vi "Send Request.vi"(8 "error in (no error)":errorcluster, 10 "ServerRequest":refnum<class "ControlPacket.lvclass">, 11 "Session in":refnum<class "Session.lvclass">) -> (0 "error out":errorcluster, 3 "Session out":refnum<class "Session.lvclass">)   [LabVIEW 2013, in "MQTT Server.lvlib" / "Session.lvclass"]
uses:
  Session.lvclass
  Control Packets/ControlPacket/ControlPacket.lvclass
  Server class/Request -- cluster.ctl
  Server class/Response -- cluster.ctl
  Session.lvclass/Session.ctl
  Server class/Server.lvclass
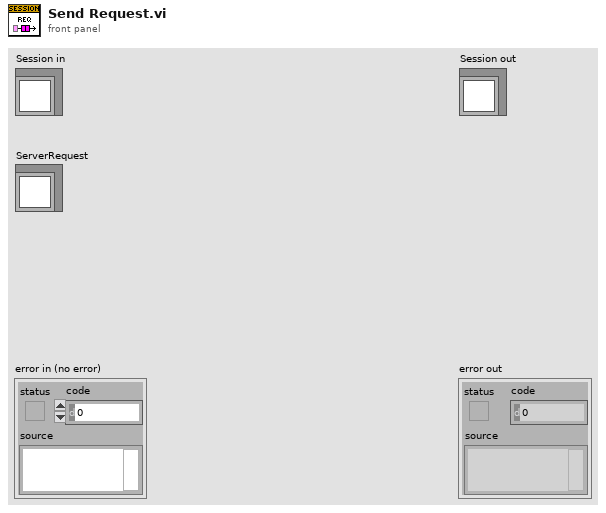
[diagram p1: front panel]
types:
  T1 = typedef "MQTT Server.lvlib/Server.lvclass/Request -- cluster.ctl" = cluster{"ServerRequest":refnum<class "ControlPacket.lvclass">, "SessionMailbox":refnum<queue>}
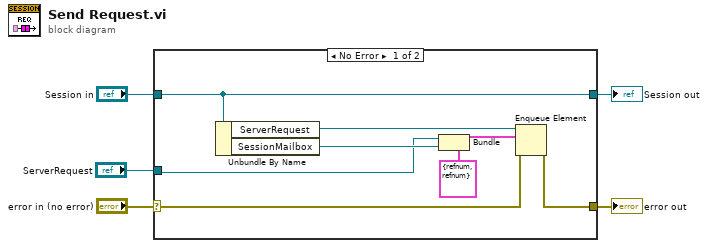
[diagram p0: block diagram]
diagram:
  n1 = case shown="No Error" "error in (no error)" {
    selector: "error in (no error)" -> [w11 w15]
    tunnel: [w10 w15] -> w4
    tunnel: [w13 w14] -> w2
    tunnel: "Session in" -> [w13 w14]
    tunnel: "ServerRequest" -> [w8 _]
    frame No Error {
      n2 = Unbundle By Name(w13) -> ("ServerRequest"=w12:refnum<queue>, "SessionMailbox"=w9:refnum<queue>)
      n3 = Bundle(cluster=T1 {"ServerRequest"=refnum, "SessionMailbox"=refnum} ("Request"), "ServerRequest"=w8, "SessionMailbox"=w9) -> (w7:T1)
      n4 = Enqueue Element(queue=w12, element=w7, error in (no error)=w11) -> (error out=w10:errorcluster)  [unwired: 1 in, 2 out]
    }
    frame Error {
    }
  }
  "error out" <- w4
  "Session out" <- w2
